vi "tcp read design inputs.vi"(8 "error in (no error)":errorcluster, 11 "listener ID in":refnum<k5>) -> (0 "error out":errorcluster, 1 "success":bool, 3 "Design Inputs":variant)   [LabVIEW 2015]
panel:
  in  "Design Inputs type":variant
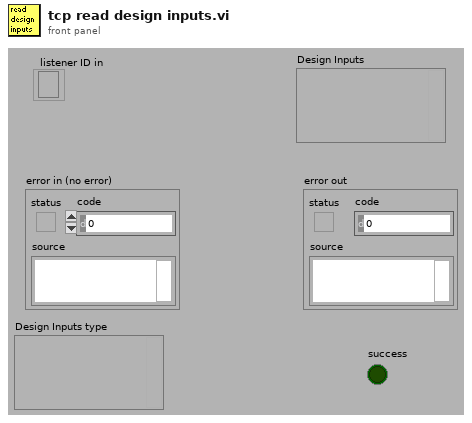
[diagram p1: front panel]
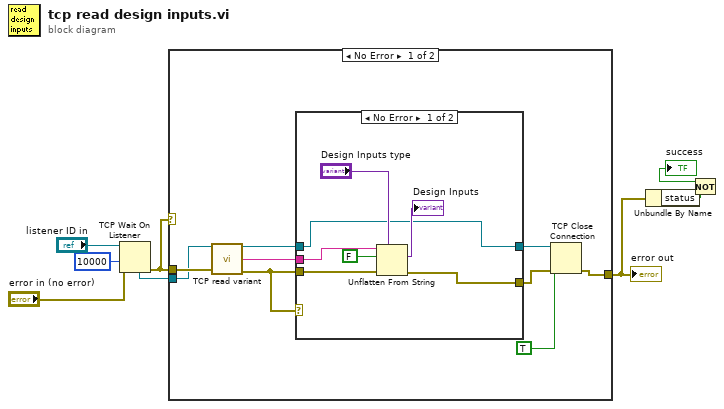
[diagram p0: block diagram]
diagram:
  n1 = TCP Wait On Listener(8:"error in (no error)", 9:10000 ("timeout ms (wait forever: -1)"), 11:"listener ID in") -> (0:w4:errorcluster, 4:w6:refnum<k5>)  [unwired: 1 in, 3 out]
  n2 = case shown="No Error" w4 {
    tunnel: w4 -> [w17 w27]
    tunnel: w6 -> [w14 _]
    tunnel: [w10 w27] -> w2
    frame No Error {
      n3 = call "TCP read variant.vi"("connection ID"=w14, "error in (no error)"=w17) -> ("connection ID out"=w13:refnum<k5>, "data out"=w16:string, "error out"=w15:errorcluster)  [unwired: 10 in, 1 out]
      n4 = case shown="No Error" w15 {
        tunnel: [w22 w25] -> w11
        tunnel: w16 -> [w21 _]
        tunnel: w15 -> [w19 w25]
        tunnel: w13 -> [w18 w26]
        tunnel: [w18 w26] -> w12
        frame No Error {
          n5 = Unflatten From String(type="Design Inputs type", binary string=w21, data includes array or string size? (T)=FALSE, error in (no error)=w19) -> (value=→"Design Inputs":variant, error out=w22:errorcluster)  [unwired: 1 in, 1 out]
        }
        frame Error {
        }
      }
      n6 = TCP Close Connection(connection ID=w12, abort (F)=TRUE, error in (no error)=w11) -> (error out=w10:errorcluster)  [unwired: 1 out]
    }
    frame Error {
    }
  }
  "error out" <- w2
  n7 = Unbundle By Name(w2) -> ("status"=w3:bool)
  n8 = Not(x=w3) -> (.not. x?=→"success":bool)
